vi "PositionSameOrNot-V2.2.vi"(2 "BlueOrGreen":dbl, 4 "Position":i32[][](array[numeric])=[[0, 1], [1, 0]]) -> (0 "SamePosition?":bool, 1 "FinalColor":dbl)   [LabVIEW 2014]
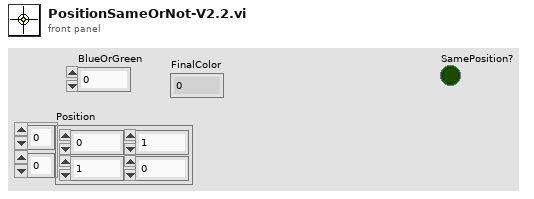
[diagram p1: front panel]
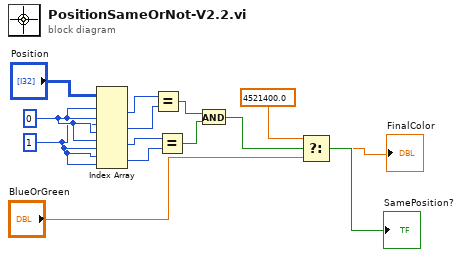
[diagram p0: block diagram]
diagram:
  w11 = 1 ("disabled index (row)")
  w12 = 0 ("index (row)")
  n1 = Index Array(array="Position", index (row) #1=w12, index (col) #1=w12, index (row) #2=w11, index (col) #2=w12, index (row) #3=w12, index (col) #3=w11, index (row) #4=w11, index (col) #4=w11) -> (element #1=w10:i32, element #2=w9:i32, element #3=w8:i32, element #4=w7:i32)
  n2 = Equal?(x=w10, y=w9) -> (x = y?=w6:bool)
  n3 = Equal?(x=w8, y=w7) -> (x = y?=w5:bool)
  n4 = And(x=w6, y=w5) -> (x .and. y?=w4:bool)
  "SamePosition?" <- w4
  n5 = Select(t=4521400.0, s=w4, f="BlueOrGreen") -> (s? t:f=→"FinalColor":dbl)
